vi "AddItems.vi"(7 "Linker.Read Info From File":T3(array[cluster]), 8 "error in (no error)":errorcluster, 9 "Settings":T1, 10 "Shallow deps?":bool, 11 "CDependencyList in":refnum<class "CDependencyList.lvclass">) -> (0 "error out":errorcluster, 1 "Debug messages":string[](array[string]), 2 "Item to enque":refnum<class "ILabVIEWItem.lvclass">[](array[class]), 3 "CDependencyList out":refnum<class "CDependencyList.lvclass">)   [LabVIEW 2020, in "DependencyInspection.lvlib" / "CDependencyList.lvclass"]
uses:
  CDependencyList.lvclass
  <vilib>/Utility/lvfile.llb/LVFileType.ctl
  ListGenerationOptions.ctl
  obj/Addons/LabVIEWObjectInterfaces.lvlibp/LabVIEWObjectInterfaces/ILabVIEWItem/ILabVIEWItem.lvclass
  obj/Addons/LabVIEWObjectFactory.lvlibp
  CDebugInfo/CDebugInfo.lvclass
  <vilib>/Utility/lvfile.llb/NI_FileType.lvlib
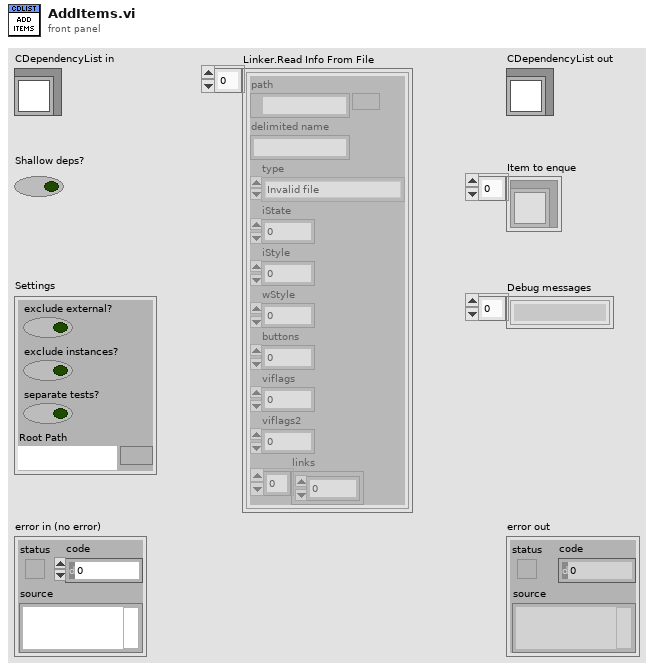
[diagram p1: front panel]
types:
  T1 = typedef "DependencyInspection.lvlib/CDependencyList.lvclass/ListGenerationOptions.ctl" = cluster{"exclude external?":bool, "exclude instances?":bool, "separate tests?":bool, "Root Path":path}
  T2 = typedef "NI_FileType.lvlib/LVFileType.ctl" = enum32{"Invalid file", "Unknown type", "Instrument", "Control", "Polymorphic VI", "Project", "Library", "LVClass", "XControl", "XNode", "Shared library", ".NET assembly", "ActiveX interface", "CIN", "Run-time menu", "Palette menu", "Help file", "LLB", "XNode Edit Dependency", "Class Private Data Control", "Statechart", "MathScript .m file", "Ladder Diagram", "LVLibp", "XNode Build Dependency"}
  T3 = cluster{"path":path, "delimited name":string, "type":T2, "iState":u32, "iStyle":u16, "wStyle":u16, "buttons":u16, "viflags":u32, "viflags2":u32, "links":u32[]}[]
  T4 = cluster{"path":path, "delimited name":string, "type":T2, "iState":u32, "iStyle":u16, "wStyle":u16, "buttons":u16, "viflags":u32, "viflags2":u32, "links":u32[]}
  T5 = typedef "LabVIEWObjectInterfaces.lvlibp/ILabVIEWItem.lvclass/RelationshipType.ctl" = enum16{"Contained", "Dependency", "Parent", "Same item", "Related", "None"}
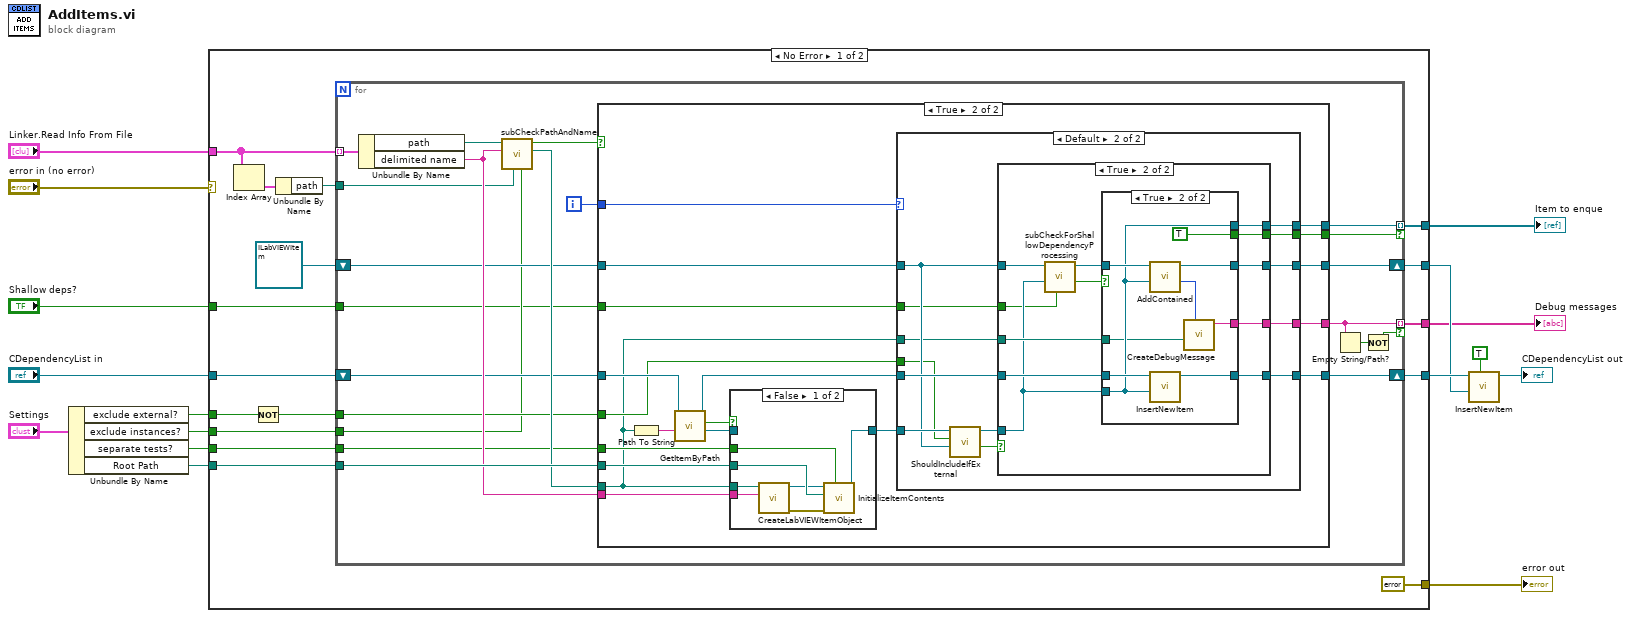
[diagram p0: block diagram]
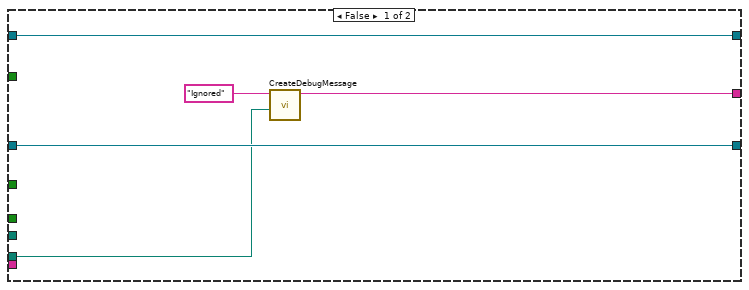
[diagram p2: hidden frame]
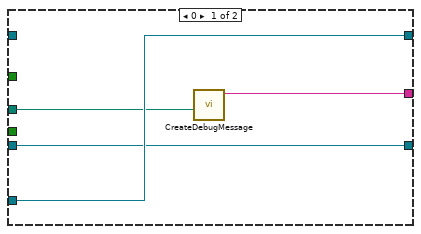
[diagram p3: hidden frame]
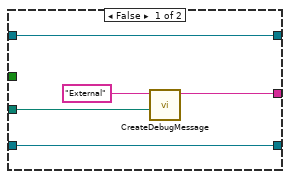
[diagram p4: hidden frame]
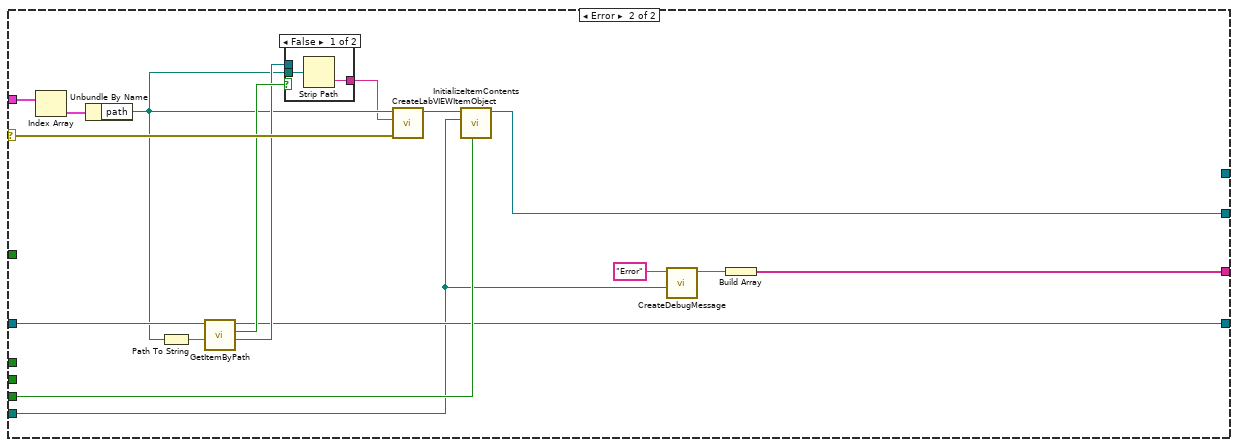
[diagram p7: hidden frame]
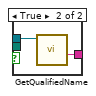
[diagram p8: hidden frame]
diagram:
  n1 = Unbundle By Name("Settings") -> ("exclude external?"=w7:bool, "exclude instances?"=w6:bool, "separate tests?"=w5:bool, "Root Path"=w4:path)
  n2 = case shown="No Error" "error in (no error)" {
    selector: "error in (no error)" -> [_ w147]
    tunnel: "Linker.Read Info From File" -> [w29 w145]
    tunnel: "CDependencyList in" -> [w32 w142]
    tunnel: [w31 w136] -> w16
    tunnel: w4 -> [w30 w133]
    tunnel: [w28 _] -> w3
    tunnel: [errorcluster {"status"=FALSE, "code"=0, "source"=""} ("error out") _] -> w13
    tunnel: w5 -> [w24 w143]
    tunnel: w6 -> [w23 _]
    tunnel: [w21 w135] -> w15
    tunnel: w7 -> [w20 _]
    tunnel: [w18 w131] -> w2
    tunnel: "Shallow deps?" -> [w17 _]
    frame No Error {
      n3 = Index Array(array=w29) -> (element=w27:T4)  [unwired: 1 in]
      n4 = Not(x=w20) -> (.not. x?=w19:bool)
      n5 = Unbundle By Name(w27) -> ("path"=w26:path)
      n6 = for {
        tunnel: w29 -> [w53] mode=indexing
        shift-right: [w50] -> w31
        shift-left: w32 -> [w44]
        tunnel: w30 -> [w51]
        tunnel: w26 -> [w46]
        tunnel: w24 -> [w43]
        tunnel: w23 -> [w38]
        shift-right: [w42] -> w21
        shift-left: refnum<class "ILabVIEWItem.lvclass"> refnum ("ILabVIEWItem out") -> [w41]
        tunnel: w19 -> [w39]
        tunnel: w17 -> [w37]
        tunnel: [w45] -> w28 mode=indexing if=w36
        tunnel: [w35] -> w18 mode=indexing if=w33
        i -> [w40]
        n7 = Unbundle By Name(w53) -> ("path"=w52:path, "delimited name"=w47:string)
        n8 = call "subCheckPathAndName.vi"("exclude instances?"=w38, "parent path"=w46, "delimited name"=w47, "path"=w52) -> ("path out"=w48:path, "path to check?"=w49:bool)  [unwired: 6 in]
        n9 = case shown="True" w49 {
          tunnel: w44 -> [w58 w74]
          tunnel: w48 -> [w54 w61]
          tunnel: w51 -> [_ w76]
          tunnel: [w58 w65] -> w50
          tunnel: w47 -> [_ w77]
          tunnel: [_ w64] -> w45
          tunnel: w43 -> [_ w75]
          tunnel: [w57 w66] -> w42
          tunnel: w41 -> [w57 w68]
          tunnel: w40 -> [_ w70]
          tunnel: w39 -> [_ w63]
          tunnel: [w56 w62] -> w35
          tunnel: w37 -> [_ w60]
          tunnel: [_ w59] -> w36
          frame False {
            n10 = call "CreateDebugMessage.vi"("Path"=w54, "Message"="Ignored") -> ("Debug message"=w56:string)  [unwired: 9 in]
          }
          frame True {
            n11 = Path To String(path=w61) -> (string=w73:string)
            n12 = call-dynamic "GetItemByPath.vi"("Path"=w73, "CDependencyList in"=w74) -> ("ILabVIEWItem"=w72:refnum<class "ILabVIEWItem.lvclass">, "key found?"=w71:bool, "CDependencyList out"=w67:refnum<class "CDependencyList.lvclass">)  [unwired: 6 in, 1 out]
            n13 = case shown="False" w71 {
              tunnel: w77 -> [w129 _]
              tunnel: w76 -> [w128 _]
              tunnel: w75 -> [w127 _]
              tunnel: w61 -> [w126 _]
              tunnel: [w123 w130] -> w69
              tunnel: w72 -> [_ w130]
              frame False {
                n14 = call "CreateLabVIEWItemObject.vi"("delimited name"=w129, "SubVI path"=w126) -> ("error out"=w124:errorcluster, "ILabVIEWItem"=w125:refnum<class "ILabVIEWItem.lvclass">)  [unwired: 8 in]
                n15 = call-dynamic "InitializeItemContents.vi"("separate test?"=w127, "error in (no error)"=w124, "Root path"=w128, "ILabVIEWItem in"=w125) -> ("ILabVIEWItem out"=w123:refnum<class "ILabVIEWItem.lvclass">)  [unwired: 6 in, 1 out]
              }
              frame True {
              }
            }
            n16 = case shown="Default" w70 {
              tunnel: [w81 w91] -> w66
              tunnel: w69 -> [w81 w90]
              tunnel: w68 -> [_ w89]
              tunnel: w67 -> [w80 w93]
              tunnel: [_ w94] -> w64
              tunnel: [w80 w92] -> w65
              tunnel: w63 -> [_ w88]
              tunnel: [w78 w85] -> w62
              tunnel: w61 -> [w79 w84]
              tunnel: w60 -> [_ w83]
              tunnel: [_ w82] -> w59
              frame 0 {
                n17 = call "CreateDebugMessage.vi"("Path"=w79) -> ("Debug message"=w78:string)  [unwired: 10 in]
              }
              frame Default {
                n18 = call-dynamic "ShouldIncludeIfExternal.vi"("Current item"=w89, "Include external?"=w88, "ILabVIEWItem in"=w90) -> ("Include?"=w86:bool, "ILabVIEWItem out"=w87:refnum<class "ILabVIEWItem.lvclass">)  [unwired: 6 in, 1 out]
                n19 = case shown="True" w86 {
                  tunnel: [_ w101] -> w94
                  tunnel: w93 -> [w98 w111]
                  tunnel: [w98 w110] -> w92
                  tunnel: [w99 w109] -> w91
                  tunnel: w89 -> [w99 w106]
                  tunnel: w87 -> [_ w104]
                  tunnel: [w95 w108] -> w85
                  tunnel: w84 -> [w96 w107]
                  tunnel: w83 -> [_ w103]
                  tunnel: [_ w100] -> w82
                  frame False {
                    n20 = call "CreateDebugMessage.vi"("Path"=w96, "Message"="External") -> ("Debug message"=w95:string)  [unwired: 9 in]
                  }
                  frame True {
                    n21 = call "subCheckForShallowDependencyProcessing.vi"("Shallow deps?"=w103, "ILabVIEWItem to enqueue"=w104, "Current ILabVIEWItem in"=w106) -> ("Process?"=w102:bool, "Current ILabVIEWItem"=w105:refnum<class "ILabVIEWItem.lvclass">)  [unwired: 7 in]
                    n22 = case shown="True" w102 {
                      tunnel: w111 -> [w112 w122]
                      tunnel: [w112 w121] -> w110
                      tunnel: [w113 w120] -> w109
                      tunnel: [_ w116] -> w108
                      tunnel: w107 -> [_ w117]
                      tunnel: w105 -> [w113 w119]
                      tunnel: w104 -> [_ w118]
                      tunnel: [_ w118] -> w101
                      tunnel: [_ TRUE] -> w100
                      frame False {
                      }
                      frame True {
                        n23 = call-dynamic "AddContained.vi"("Item to contain"=w118, "ILabVIEWItem in"=w119) -> ("Relationship type"=w114:T5, "ILabVIEWItem out"=w120:refnum<class "ILabVIEWItem.lvclass">)  [unwired: 7 in, 1 out]
                        n24 = call-dynamic "InsertNewItem.vi"("ILabVIEWItem in"=w118, "CDependencyList in"=w122) -> ("CDependencyList out"=w121:refnum<class "CDependencyList.lvclass">)  [unwired: 7 in, 2 out]
                        n25 = call "CreateDebugMessage.vi"("Relationship type"=w114, "Path"=w117) -> ("Debug message"=w116:string)  [unwired: 9 in]
                      }
                    }
                  }
                }
              }
            }
          }
        }
        n26 = Empty String/Path?(string/path=w35) -> (empty?=w34:bool)
        n27 = Not(x=w34) -> (.not. x?=w33:bool)
      }
    }
    frame Error {
      n28 = Index Array(array=w145) -> (element=w146:T4)  [unwired: 1 in]
      n29 = Unbundle By Name(w146) -> ("path"=w138:path)
      n30 = Path To String(path=w138) -> (string=w141:string)
      n31 = call-dynamic "GetItemByPath.vi"("Path"=w141, "CDependencyList in"=w142) -> ("ILabVIEWItem"=w139:refnum<class "ILabVIEWItem.lvclass">, "key found?"=w140:bool, "CDependencyList out"=w136:refnum<class "CDependencyList.lvclass">)  [unwired: 6 in, 1 out]
      n32 = case shown="False" w140 {
        tunnel: w139 -> [_ w151]
        tunnel: w138 -> [w149 _]
        tunnel: [w148 w150] -> w137
        frame False {
          n33 = Strip Path(path=w149) -> (name=w148:string)  [unwired: 1 out]
        }
        frame True {
          n34 = call-dynamic "GetQualifiedName.vi"("ILabVIEWItem in"=w151) -> ("Qualified name"=w150:string)  [unwired: 8 in, 2 out]
        }
      }
      n35 = call "CreateLabVIEWItemObject.vi"("error in (no error)"=w147, "delimited name"=w137, "SubVI path"=w138) -> ("ILabVIEWItem"=w144:refnum<class "ILabVIEWItem.lvclass">)  [unwired: 7 in, 1 out]
      n36 = call-dynamic "InitializeItemContents.vi"("separate test?"=w143, "Root path"=w133, "ILabVIEWItem in"=w144) -> ("ILabVIEWItem out"=w135:refnum<class "ILabVIEWItem.lvclass">)  [unwired: 7 in, 1 out]
      n37 = call "CreateDebugMessage.vi"("Path"=w133, "Message"="Error") -> ("Debug message"=w132:string)  [unwired: 9 in]
      n38 = Build Array(w132) -> (w131:string[])
    }
  }
  "error out" <- w13
  "Item to enque" <- w3
  "Debug messages" <- w2
  n39 = call-dynamic "InsertNewItem.vi"("Replace?"=TRUE, "ILabVIEWItem in"=w15, "CDependencyList in"=w16) -> ("CDependencyList out"=→"CDependencyList out":refnum<class "CDependencyList.lvclass">)  [unwired: 6 in, 2 out]
